vi "Server Manager Test.vi"() -> ()   [LabVIEW 2017, in "Echo Broadcast Test With Server Manager.lvlib"]
uses:
  Echo Broadcast Test With Server Manager.lvlib
  WebSocket Actor/WebSocket Server Manager/WebSocket Server Manager.lvclass
  C:/Program Files (x86)/National Instruments/LabVIEW 2017/vi.lib/ActorFramework/Actor/Actor.lvclass
  <vilib>/ActorFramework/Actor/Actor.lvclass
panel:
  out "error out":errorcluster
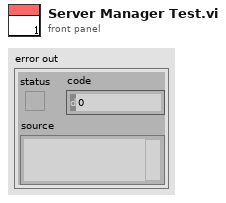
[diagram p1: front panel]
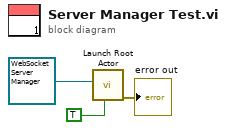
[diagram p0: block diagram]
diagram:
  n1 = call <vilib>:"Launch Root Actor.vi"("Open Actor Core front panel? (F)"=TRUE, "Actor"=refnum<class "WebSocket Server Manager.lvclass"> refnum ("WebSocket Actors.lvlib:WebSocket Server Manager.lvclass")) -> ("error out"=→"error out":errorcluster)  [unwired: 8 in, 1 out]
